vi "Lian_Lab06_II.vi"() -> ()   [LabVIEW 2020]
uses:
  <vilib>/DAQmx/read.llb/DAQmx Read (Analog Wfm 1Chan NSamp).vi
  <vilib>/DAQmx/create/channels.llb/DAQmx Create Channel (AI-Voltage-Basic).vi
  <vilib>/DAQmx/configure/timing.llb/DAQmx Timing (Sample Clock).vi
  <vilib>/DAQmx/miscellaneous.llb/DAQmx Fill In Error Info.vi
panel:
  in  "?":bool
  in  "number of samples per channel":i32=20
  out "Waveform Chart":waveform(dbl)(graph)
  in  "sample mode":i32(ring)=10123 items=["Finite Samples"=10178, "Continuous Samples"=10123, "Hardware Timed Single Point"=12522]
  in  "rate":dbl=200000.0 format="%0.2f"
  in  "samples per channel":i32=10000
  in  "input terminal configuration":i32(ring)=10106 items=["Default"=-1, "RSE"=10083, "NRSE"=10078, "Differential"=10106, "Pseudodifferential"=12529]
  in  "maximum value":dbl=10.0 format="%0.2f"
  in  "minimum value":dbl=-10.0 format="%0.2f"
  in  "physical channels":tag="myDAQ1/ai0"
  # "Part II. Continuous Acquisition"
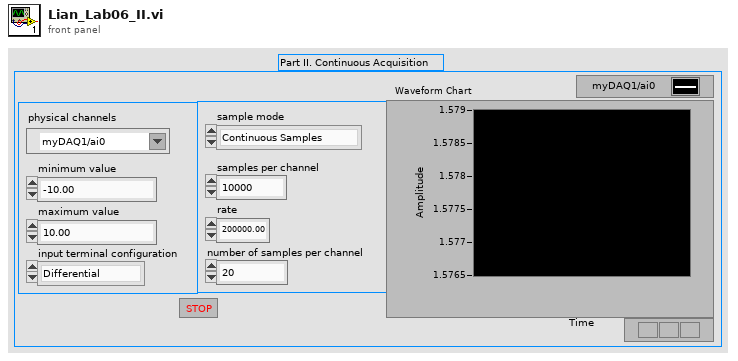
[diagram p1: front panel]
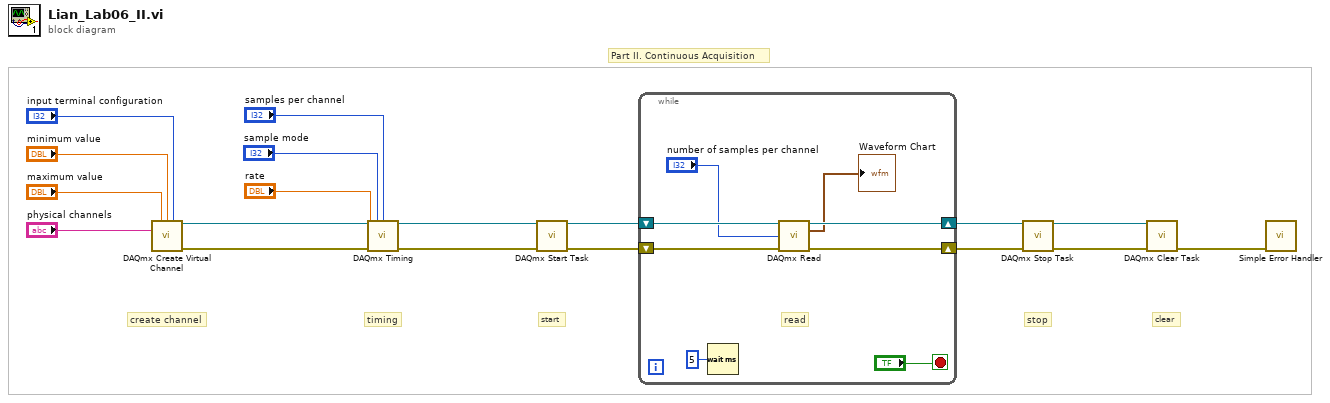
[diagram p0: block diagram]
diagram:
  # "Part II. Continuous Acquisition"
  # "clear"
  # "stop"
  # "start"
  # "timing"
  # "create channel"
  n1 = call-poly <vilib>:"DAQmx Create Virtual Channel.vi"("maximum value"="maximum value", "minimum value"="minimum value", "input terminal configuration"="input terminal configuration", "physical channels"="physical channels") -> ("task out"=w12:refnum<k21>, "error out"=w7:errorcluster)  [unwired: 10 in]
  n2 = call-poly <vilib>:"DAQmx Timing.vi"("task/channels in"=w12, "sample mode"="sample mode", "samples per channel"="samples per channel", "rate"="rate", "error in"=w7) -> ("task out"=w11:refnum<k21>, "error out"=w6:errorcluster)  [unwired: 9 in]
  n3 = call <vilib>:"DAQmx Start Task.vi"("task/channels in"=w11, "error in"=w6) -> ("task out"=w10:refnum<k21>, "error out"=w5:errorcluster)  [unwired: 12 in]
  n4 = while {
    shift-right: [w25] -> w9
    shift-left: w10 -> [w26]
    shift-right: [w23] -> w4
    shift-left: w5 -> [w24]
    stop <- "?" stop-if-true
    # "read"
    n5 = Wait (ms)(milliseconds to wait=u32 5) -> ()  [unwired: 1 out]
    n6 = call-poly <vilib>:"DAQmx Read.vi"("task/channels in"=w26, "number of samples per channel"="number of samples per channel", "error in"=w24) -> ("task out"=w25:refnum<k21>, "data"=→"Waveform Chart":waveform(dbl), "error out"=w23:errorcluster)  [unwired: 10 in]
  }
  n7 = call <vilib>:"DAQmx Stop Task.vi"("task/channels in"=w9, "error in"=w4) -> ("task out"=w8:refnum<k21>, "error out"=w3:errorcluster)  [unwired: 12 in]
  n8 = call <vilib>:"DAQmx Clear Task.vi"("task in"=w8, "error in"=w3) -> ("error out"=w2:errorcluster)  [unwired: 13 in]
  n9 = call <vilib>:"Simple Error Handler.vi"("error in (no error)"=w2) -> ()  [unwired: 4 in, 5 out]
